vi "Revision Query.vi"(8 "error in (no error)":errorcluster, 11 "VISA resource name":refnum<visa-resource-name>) -> (0 "error out":errorcluster, 1 "Instrument Driver Revision":string, 2 "Identification":string, 3 "VISA resource name out":refnum<visa-resource-name>)   [LabVIEW 2018, in "LTB-1.lvlib" / "3150.lvlib"]
doc: "This VI queries the current instrument driver revision and unique identification of devices over the system interface."
uses:
  3150.lvlib
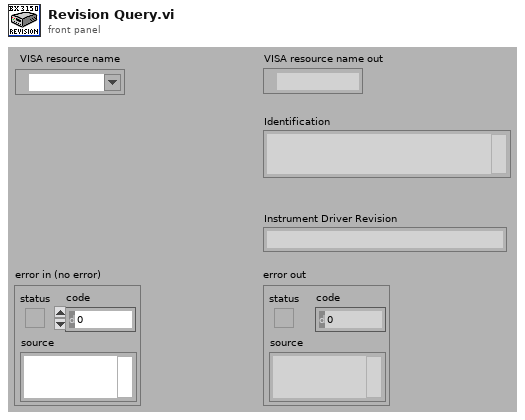
[diagram p1: front panel]
types:
  T1 = enum32{"invalid app kind", "Development System", "Run Time System", "Student Edition", "Embedded LabVIEW", "Evaluation", "Custom"}
  T2 = cluster{"Major":u16, "Minor":u16, "Fix":u16, "Build":u16}
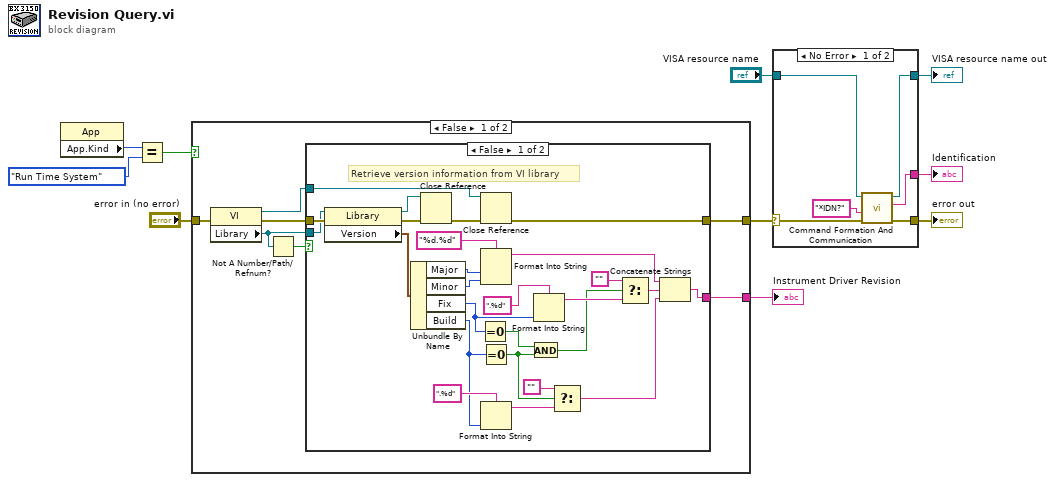
[diagram p0: block diagram]
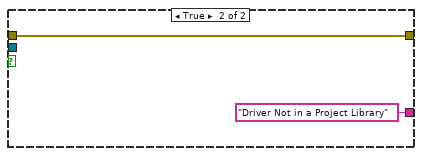
[diagram p2: hidden frame]
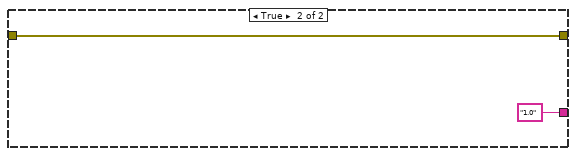
[diagram p3: hidden frame]
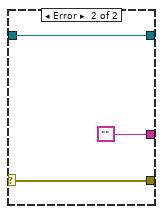
[diagram p4: hidden frame]
diagram:
  n1 = property class="App"() -> ("App.Kind"=w6:T1)  [unwired: 2 in, 2 out]
  n2 = Equal?(x=w6, y=T1."Run Time System" ("Application:Kind")) -> (x = y?=w4:bool)
  n3 = case shown="False" w4 {
    tunnel: [w13 "1.0"] -> w1
    tunnel: [w12 w46] -> w2
    tunnel: "error in (no error)" -> [w11 w46]
    frame False {
      n4 = property class="VI"(error in=w11) -> (reference out=w17:refnum<vi>, error out=w16:errorcluster, "Library"=w15:refnum<vi>)  [unwired: 1 in]
      n5 = Not A Number/Path/Refnum?(number/path/refnum=w15) -> (NaN/Path/Refnum?=w14:bool)
      n6 = case shown="False" w14 {
        tunnel: w17 -> [w40 _]
        tunnel: w16 -> [w25 w45]
        tunnel: [w20 w45] -> w12
        tunnel: [w19 "Driver Not in a Project Library"] -> w13
        tunnel: w15 -> [w18 _]
        frame False {
          # "Retrieve version information from VI library"
          n7 = property class="Library"(reference=w18, error in=w25) -> (reference out=w42:refnum<vi>, error out=w43:errorcluster, "Version"=w39:T2)
          n8 = Unbundle By Name(w39) -> ("Major"=w28:u16, "Minor"=w27:u16, "Fix"=w24:u16, "Build"=w26:u16)
          n9 = Close Reference(reference=w42, error in (no error)=w43) -> (error out=w41:errorcluster)
          n10 = Equal To 0?(x=w24) -> (x = 0?=w23:bool)
          n11 = Close Reference(reference=w40, error in (no error)=w41) -> (error out=w20:errorcluster)
          n12 = Format Into String(format string="%d.%d", w28, w27) -> (resulting string=w34:string)  [unwired: 2 in, 1 out]
          n13 = Equal To 0?(x=w26) -> (x = 0?=w22:bool)
          n14 = Format Into String(format string=".%d", w26) -> (resulting string=w32:string)  [unwired: 2 in, 1 out]
          n15 = And(x=w23, y=w22) -> (x .and. y?=w21:bool)
          n16 = Format Into String(format string=".%d", w24) -> (resulting string=w36:string)  [unwired: 2 in, 1 out]
          n17 = Select(t="", s=w22, f=w32) -> (s? t:f=w29:string)
          n18 = Select(t="", s=w21, f=w36) -> (s? t:f=w33:string)
          n19 = Concatenate Strings(w34, w33, w29) -> (w19:string)
        }
        frame True {
        }
      }
    }
    frame True {
    }
  }
  "Instrument Driver Revision" <- w1
  n20 = case shown="No Error" w2 {
    selector: w2 -> [w53 w56]
    tunnel: [w52 w56] -> w7
    tunnel: [w51 w55] -> w8
    tunnel: "VISA resource name" -> [w50 w55]
    tunnel: [w48 ""] -> w10
    frame No Error {
      n21 = call "Command Formation And Communication.vi"("error in (no error)"=w53, "Command"="*IDN?", "VISA resource name"=w50) -> ("error out"=w52:errorcluster, "Response"=w48:string, "VISA resource name out"=w51:refnum<visa-resource-name>)  [unwired: 1 in, 5 out]
    }
    frame Error {
    }
  }
  "Identification" <- w10
  "VISA resource name out" <- w8
  "error out" <- w7
